vi "High Frequency UI.vi"(11 "Event":refnum<event-registration>) -> ()   [LabVIEW 2012]
uses:
  Data/cPAS Data.lvclass
  Reusable/PAS/Data/Main/Read CellData.vi
  Reusable/PAS/Data/Cell/Read timeData.vi
  Reusable/PAS/Data/Cell/Read lasDiodeData.vi
  Reusable/PAS/Data/Cell/Read Fitted Data.vi
  Reusable/PAS/Data/Cell/Read freqData.vi
  Reusable/PAS/Data/Cell/Read f0.vi
  Reusable/PAS/Data/Cell/Read Q.vi
  Reusable/PAS/Data/Cell/PAS Cell Data.lvclass
panel:
  in  "log_lin":bool
  out "Q":sgl format="%.2f"
  out "f0":sgl
  in  "cell":T1(ring)
  out "micTime":waveform(i16)(graph) caption="Time Domain"
  out "micFreq":cluster{i32, dbl, "Y":sgl[]}[](graph) caption="Frequency Domain"
  out "diodeTime":waveform(i16)(graph) caption="Photodiode Time Domain"
  out "lastCal":timestamp caption="Last Speaker Calibration" format="%<%H:%M:%S>T"
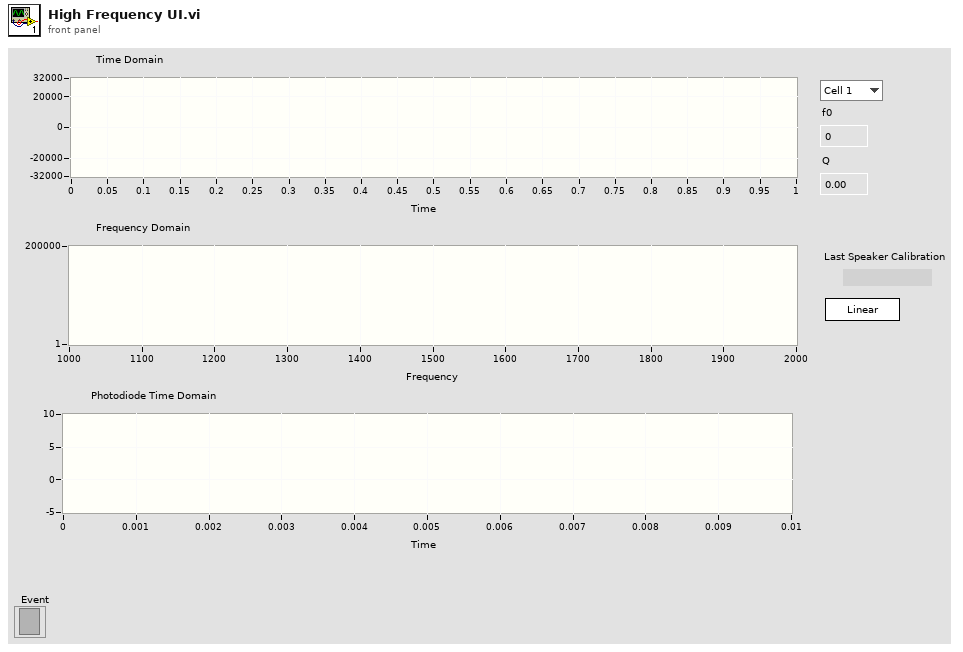
[diagram p1: front panel]
types:
  T1 = enum16{"Cell 1", "Cell 2", "Cell 3", "Cell 4", "Cell 5"}
  T2 = cluster{"Read Access":enum8{"Allowed", "Required", "None"}, "Write Access":enum8{"Allowed", "Required", "None"}}
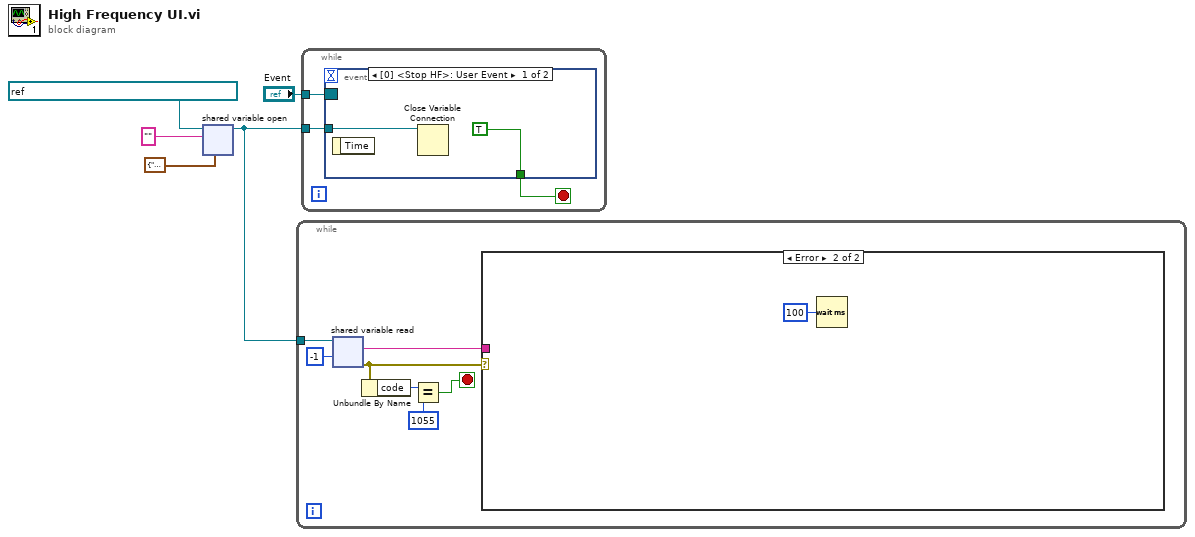
[diagram p0: block diagram]
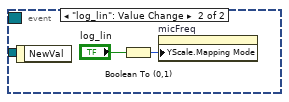
[diagram p2: hidden frame]
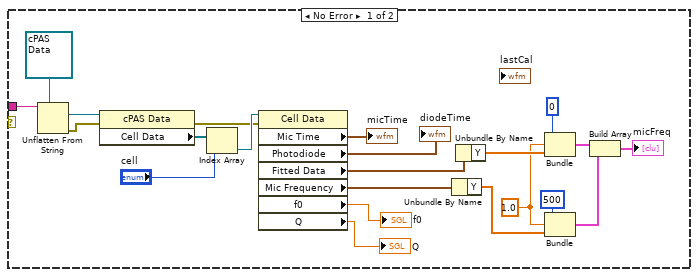
[diagram p3: hidden frame]
diagram:
  n1 = shared-variable-open(refnum<k21> "ni.var.psp://rt pxi target/PAS_Var/Data" ("shared variable refnum in"), "", T2 {"Read Access"=enum."Allowed", "Write Access"=enum."None"} ("access")) -> (w4:refnum<k21>)  [unwired: 1 in, 1 out]
  n2 = while {
    tunnel: w4 -> [w12]
    stop <- w6 stop-if-true
    n3 = shared-variable-read(w12, -1 ("timeout ms")) -> (w9:errorcluster, w10:string)  [unwired: 1 in, 3 out]
    n4 = Unbundle By Name(w9) -> ("code"=w8:i32)
    n5 = Equal?(x=w8, y=1055) -> (x = y?=w6:bool)
    n6 = case shown="Error" w9 {
      tunnel: w10 -> [w14 _]
      frame No Error {
        w26 = 1.0
        n7 = Unflatten From String(type=refnum<class "cPAS Data.lvclass"> refnum ("PAS Data.lvclass"), binary string=w14) -> (value=w33:refnum<class "cPAS Data.lvclass">, error out=w13:errorcluster)  [unwired: 3 in, 1 out]
        n8 = property class="cPAS Data"(reference=w33, error in=w13) -> (error out=w29:errorcluster, "Cell Data"=w32:refnum<class "PAS Cell Data.lvclass">[])  [unwired: 1 out]
        n9 = Index Array(array=w32, index="cell") -> (element=w30:refnum<class "PAS Cell Data.lvclass">)
        n10 = property class="Cell Data"(reference=w30, error in=w29) -> ("Mic Time"=→"micTime":waveform(i16), "Photodiode"=→"diodeTime":waveform(i16), "Fitted Data"=w21:waveform(sgl), "Mic Frequency"=w20:waveform(sgl), "f0"=→"f0":sgl, "Q"=→"Q":sgl)  [unwired: 2 out]
        n11 = Unbundle By Name(w20) -> ("Y"=w28:sgl[])
        n12 = Unbundle By Name(w21) -> ("Y"=w27:sgl[])
        n13 = Bundle(0, w26, "Y"=w27) -> (w24:cluster{i32, dbl, "Y":sgl[]})  [unwired: 1 in]
        n14 = Bundle(500, w26, "Y"=w28) -> (w23:cluster{i32, dbl, "Y":sgl[]})  [unwired: 1 in]
        n15 = Build Array(w24, w23) -> (→"micFreq":cluster{i32, dbl, "Y":sgl[]}[])
      }
      frame Error {
        n16 = Wait (ms)(milliseconds to wait=u32 100) -> ()  [unwired: 1 out]
      }
    }
  }
  n17 = while {
    tunnel: w4 -> [w38]
    tunnel: "Event" -> [w37]
    stop <- w36 stop-if-true
    n18 = event shown="[0] <Stop HF>: User Event" {
      selector: w37 -> [_ _]
      dyn-events: _ -> [_ _]
      timeout: _ -> [_ _]
      tunnel: w38 -> [w40 _]
      tunnel: [TRUE _] -> w36
      event User Event {
        n19 = event-data() -> ()  [unwired: 1 in, 1 out]
        n20 = Close Variable Connection(11:w40) -> ()  [unwired: 1 in, 1 out]
      }
      event "log_lin": Value Change {
        n21 = event-data() -> ()  [unwired: 1 in, 1 out]
        n22 = Boolean To (0,1)(Boolean="log_lin") -> (0, 1=w41:i16)
        n23 = property on="micFreq" class="WFGraph (strict)"("YScale.Mapping Mode"=w41) -> ()  [unwired: 2 in, 2 out]
      }
    }
  }
